vi "Command Query.vi"(8 "error in (no error)":errorcluster, 9 "Delay (ms)":u32=5, 10 "Command":string, 11 "MSOX6004 in":refnum<class "MSOX6004.lvclass">) -> (0 "error out":errorcluster, 2 "Response":string, 3 "MSOX6004 out":refnum<class "MSOX6004.lvclass">)   [LabVIEW 2018, in "MSOX6004.lvlib" / "MSOX6004.lvclass"]
uses:
  MSOX6004.lvclass
  MSOX6004.lvclass/MSOX6004.ctl
  <instrlib>/Keysight InfiniiVision/Keysight InfiniiVision.lvlib
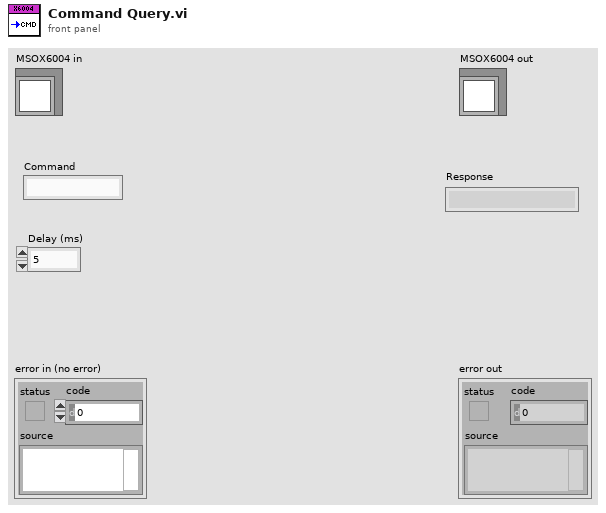
[diagram p1: front panel]
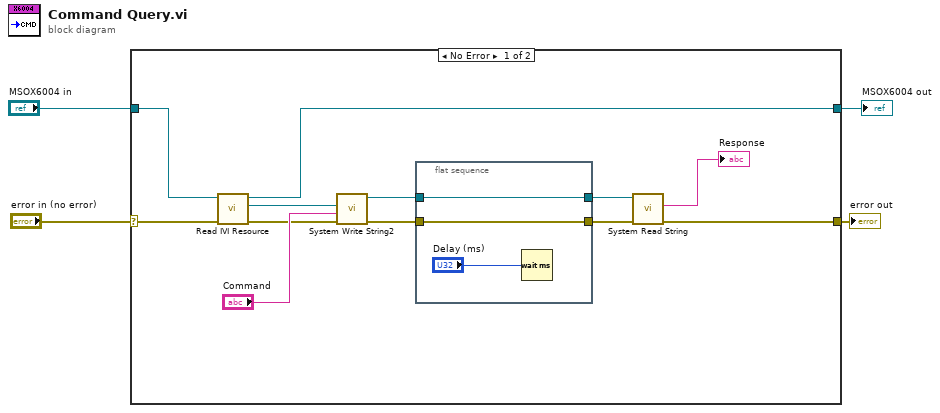
[diagram p0: block diagram]
diagram:
  n1 = case shown="No Error" "error in (no error)" {
    selector: "error in (no error)" -> [w16 w21]
    tunnel: [w5 w21] -> w3
    tunnel: [w7 w20] -> w1
    tunnel: "MSOX6004 in" -> [w15 w20]
    frame No Error {
      n2 = call "Read IVI Resource.vi"("error in (no error)"=w16, "MSOX6004 in"=w15) -> ("error out"=w8:errorcluster, "IVI Resource"=w14:refnum<k15>, "MSOX6004 out"=w7:refnum<class "MSOX6004.lvclass">)  [unwired: 7 in]
      n3 = call <instrlib>:"System Write String2.vi"("error in (no error)"=w8, "Data"="Command", "instrument handle"=w14) -> ("error out"=w9:errorcluster, "instrument handle out"=w11:refnum<k15>)  [unwired: 7 in]
      n4 = flat-sequence {
        tunnel: [w19] -> w12
        tunnel: w11 -> [w19]
        tunnel: [w17] -> w10
        tunnel: w9 -> [w17]
        frame #0 {
          n5 = Wait (ms)(milliseconds to wait="Delay (ms)") -> ()  [unwired: 1 out]
        }
      }
      n6 = call <instrlib>:"System Read String.vi"("error in (no error)"=w10, "instrument handle"=w12) -> ("error out"=w5:errorcluster, "Val"=→"Response":string)  [unwired: 7 in, 1 out]
    }
    frame Error {
    }
  }
  "error out" <- w3
  "MSOX6004 out" <- w1
